vi "MDF4 Write Data to Stream (Double).vi"(8 "Error In":errorcluster, 9 "Data":dbl, 10 "Channel Index":u32, 11 "Stream Reference in":i64) -> (0 "Error Out":errorcluster, 3 "Stream Reference out":i64)   [LabVIEW 2019, in "MD4Logger Engine.lvlib"]
uses:
  MD4Logger Engine.lvlib
  <vilib>/Utility/error.llb/Error Cluster From Error Code.vi
  <vilib>/ErrorRing/Error Ring.xnode
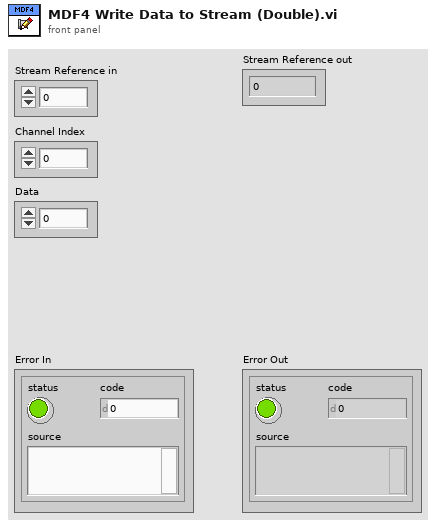
[diagram p1: front panel]
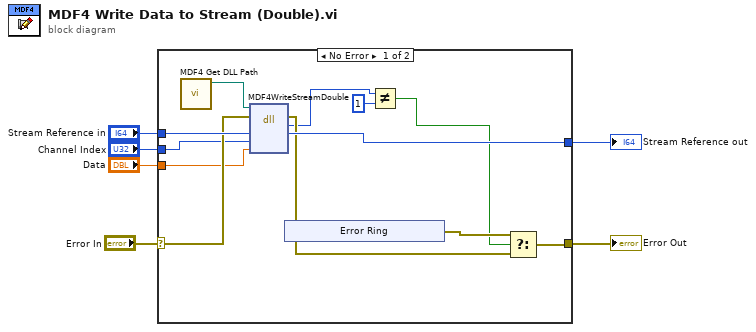
[diagram p0: block diagram]
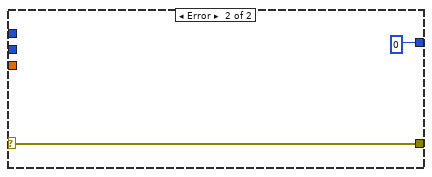
[diagram p2: hidden frame]
diagram:
  n1 = case shown="No Error" "Error In" {
    selector: "Error In" -> [w17 w25]
    tunnel: "Stream Reference in" -> [w18 _]
    tunnel: [w13 w25] -> w4
    tunnel: [w16 i64 0 ("m4")] -> w3
    tunnel: "Channel Index" -> [w15 _]
    tunnel: "Data" -> [w11 _]
    frame No Error {
      n2 = call "MDF4 Get DLL Path.vi"() -> ("DLL Path Out"=w7:path)  [unwired: 11 in]
      n3 = dll-call lib="C:/Thomas/SourceTree/ADAS-RP/logger/plugins/ADAS_MDF4/src/PE/SubVIs/MDF4 API/Low-Level API/DLL/MDF4 Wrapper.dll" fn="MDF4WriteStreamDouble"(path in=w7, error in=w17, "DStream"=w18, "channel_index"=w15, "data"=w11) -> (error out=w12:errorcluster, "return type"=w9:i32, "DStream"=w16:i64)  [unwired: 3 in, 1 out]
      n4 = xnode "Error Ring"() -> ("error out"=w14:errorcluster)
      n5 = Not Equal?(x=w9, y=1) -> (x != y?=w8:bool)
      n6 = Select(t=w14, s=w8, f=w12) -> (s? t:f=w13:errorcluster)
    }
    frame Error {
    }
  }
  "Error Out" <- w4
  "Stream Reference out" <- w3
